vi "Test Return Test Case Result for Parametrized Case.vi"(11 "Test Case In":refnum<class "Parameterized Test Case Test.lvclass">) -> (0 "error out":errorcluster, 3 "Test Case Out":refnum<class "Parameterized Test Case Test.lvclass">)   [LabVIEW 2020, in "Parameterized Test Case Test.lvclass"]
uses:
  Parameterized Test Case Test.lvclass
  C:/Program Files/National Instruments/LabVIEW 2024/vi.lib/Astemes/LUnit/Test Case.lvclass
  <vilib>/Astemes/LUnit/Test Case.lvclass/Test Case.ctl
  399136ac-e113-4bca-be3a-8dde4e32c814.vi
  <vilib>/Astemes/LUnit/Palette/Pass If.vi
  <vilib>/Astemes/LUnit/Core/LUnit Test Case/Private/Append Fail Result.vi
  <vilib>/Astemes/LUnit/Core/LUnit Test Case/Private/Append Pass Result.vi
  <vilib>/Astemes/LUnit/Core/LUnit Test Case/Private/Run In UI.vi
  <vilib>/Utility/error.llb/Clear Errors.vi
  source/Parameterized Test Case/Parameterized Test Case.lvclass
  <vilib>/Astemes/LUnit/Test Suite.lvclass
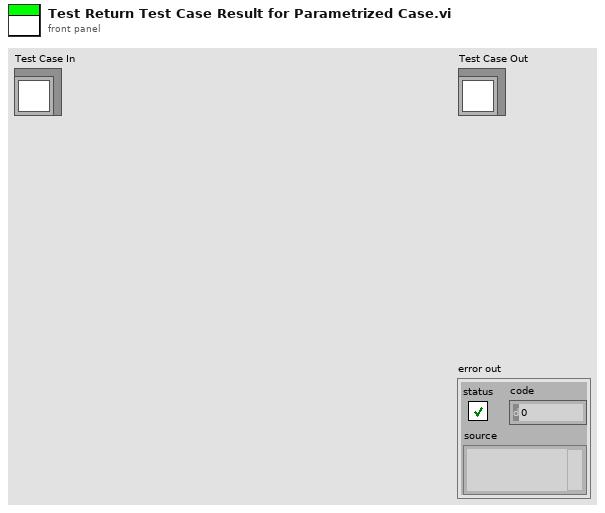
[diagram p1: front panel]
types:
  T1 = cluster{"Name":string, "Description":string, "Status":enum16{"", "Passed", "Failed", "Error", "Skipped", "Setup Error", "Broken", "Teardown Error"}, "Result Type":enum16{"Test Case", "Test Suite", "Test Run", "Pass", "Fail", "Skip", "Pass if", "Fail if", "Pass if Error", "Fail if Error", "Pass if Equal", "Fail if Equal"}, "Execution Time":dbl, "Data":cluster{"Expected":variant, "Actual":variant, "Delta":variant}}[]
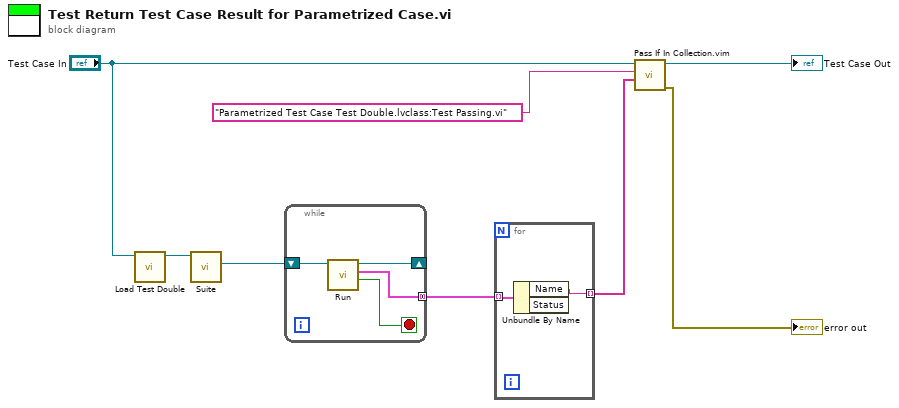
[diagram p0: block diagram]
diagram:
  n1 = call "Load Test Double.vi"("Parameterized Test Case Test in"="Test Case In") -> ("Parameterized Test Case out"=w1:refnum<class "Parameterized Test Case.lvclass">)  [unwired: 9 in, 1 out]
  n2 = call-dynamic "Suite.vi"("Parameterized Test Case In"=w1) -> ("LUnit Test Suite Out"=w5:refnum<class "Test Suite.lvclass">)  [unwired: 8 in, 2 out]
  n3 = while {
    tunnel: [w12] -> w4 mode=concatenating
    shift-right: [w10] -> _
    shift-left: w5 -> [w11]
    stop <- w9 stop-if-true
    n4 = call-dynamic "Run.vi"("LUnit Test Suite In"=w11) -> ("Done?"=w9:bool, "Results"=w12:T1, "LUnit Test Suite In 2"=w10:refnum<class "Test Suite.lvclass">)  [unwired: 7 in, 1 out]
  }
  n5 = for {
    tunnel: w4 -> [w14] mode=indexing
    tunnel: [w13] -> w3 mode=indexing
    n6 = Unbundle By Name(w14) -> ("Name"=w13:string)  [unwired: 1 out]
  }
  n7 = call "Pass If In Collection.vim"("Collection"=w3, "Expected Element"="Parametrized Test Case Test Double.lvclass:Test Passing.vi" ("String"), "LUnit Test Case In"="Test Case In") -> ("error out"=→"error out":errorcluster, "LUnit Test Case Out"=→"Test Case Out":refnum<class "Parameterized Test Case Test.lvclass">)  [unwired: 7 in]
